vi "CAN_HV_subvi_set.vi"(2 "IP adress HV2":string="1_0_0", 3 "HV Cluster":T1={"HV Power On/Off"=[], "Set Voltage"=[], "HV Tolerance (%)"=1.0}, 4 "IP adress HV1":string="0_0_0") -> (0 "error out":errorcluster, 1 "handle":i32)   [LabVIEW 2012]
uses:
  Program Files/CAEN/HV/CAENHVWrapper/labview/CAENHVWrapper/CAENHVWrapper.lvlib
panel:
  out "Channel On/Off":bool[](array[boolean])
  out "Voltage":string[](array[string])
  out "IP adress used":string
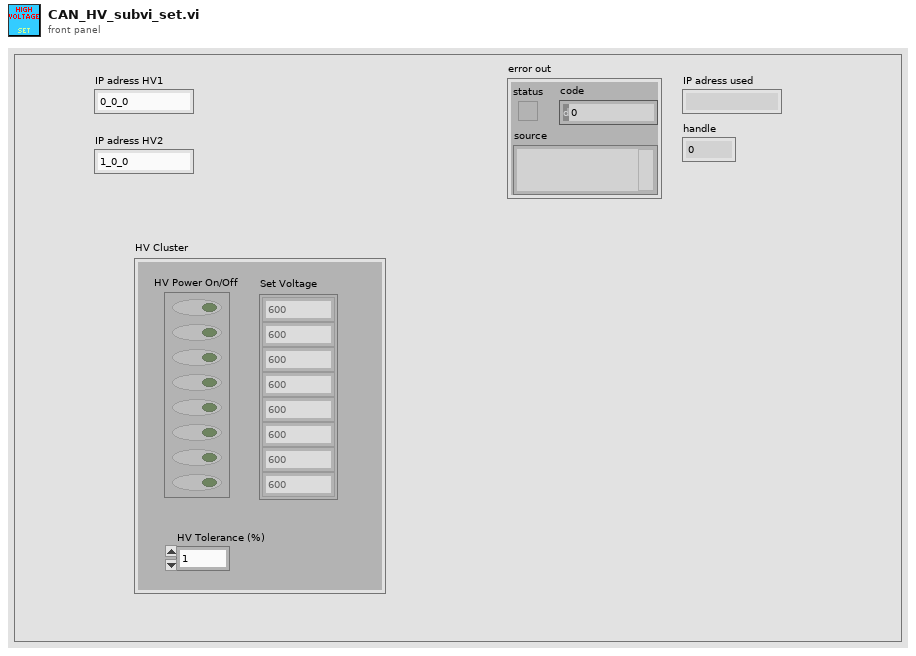
[diagram p1: front panel]
types:
  T1 = cluster{"HV Power On/Off":bool[], "Set Voltage":string[], "HV Tolerance (%)":dbl}
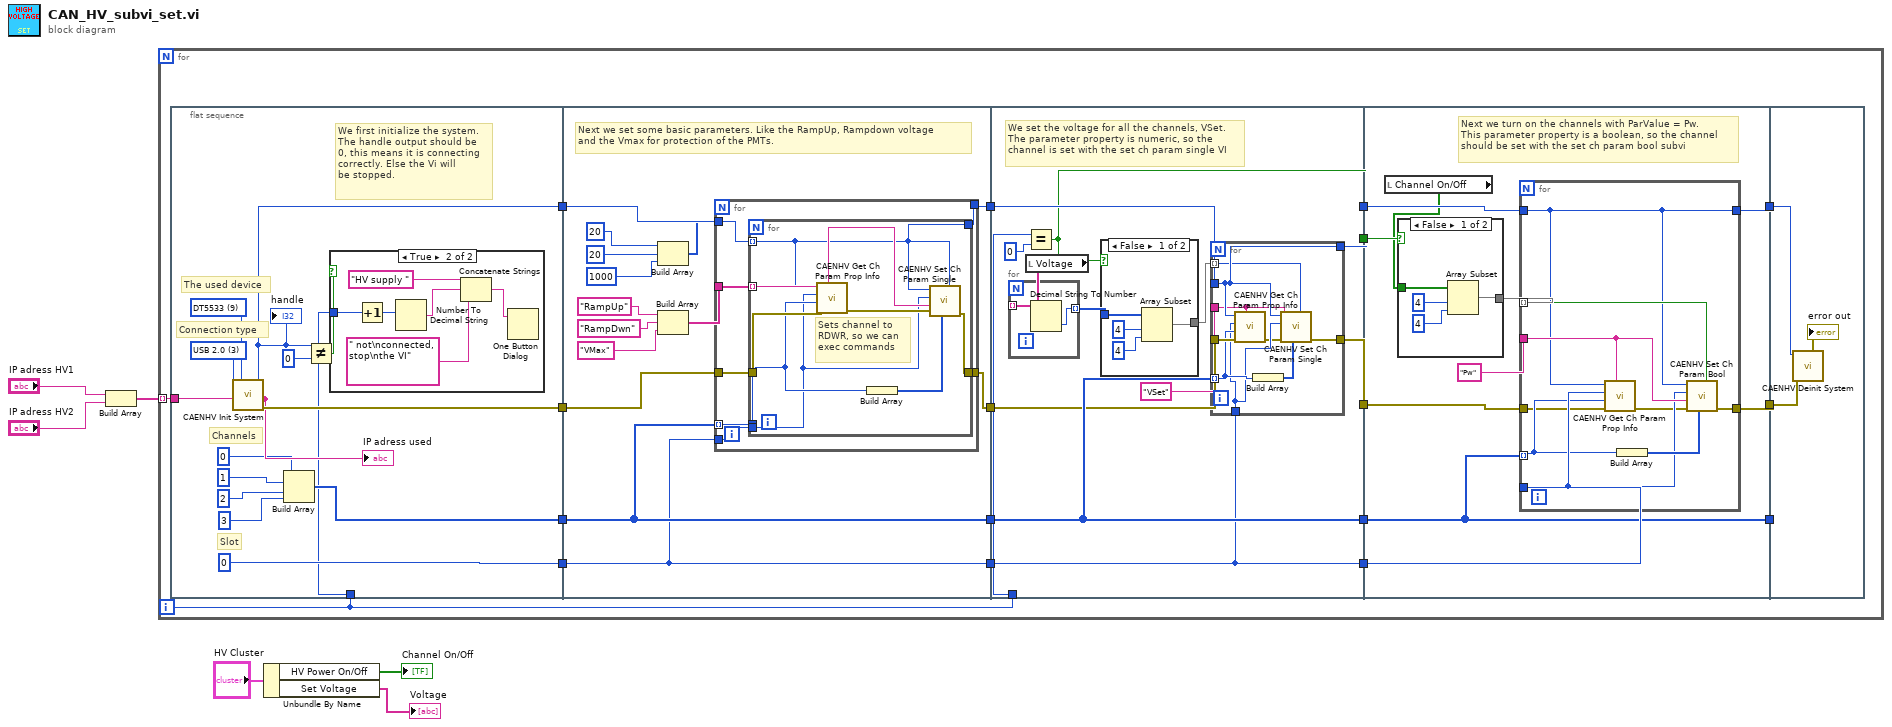
[diagram p0: block diagram]
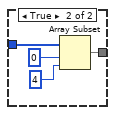
[diagram p3: hidden frame]
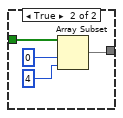
[diagram p4: hidden frame]
diagram:
  n1 = Build Array("IP adress HV1", "IP adress HV2") -> (w4:string[])
  n2 = for {
    tunnel: w4 -> [w12] mode=indexing
    i -> [w7]
    n3 = flat-sequence {
      tunnel: [w36] -> w24
      tunnel: [w32] -> w23
      tunnel: [w33] -> w22
      tunnel: [0] -> w21
      tunnel: w12 -> [w31]
      tunnel: w7 -> [w25]
      tunnel: w24 -> [w56]
      tunnel: w23 -> [w58]
      tunnel: [w57] -> w20
      tunnel: w22 -> [w50]
      tunnel: w21 -> [w49]
      tunnel: [w50] -> w19
      tunnel: [w49] -> w18
      tunnel: [w55] -> w17
      tunnel: w20 -> [w88]
      tunnel: [w87] -> w16
      tunnel: [w84] -> w15
      tunnel: [w86] -> w14
      tunnel: [w85] -> w13
      tunnel: w19 -> [w85]
      tunnel: w18 -> [w84]
      tunnel: w17 -> [w83]
      tunnel: [w79] -> w11
      tunnel: w7 -> [w78]
      tunnel: w16 -> [w116]
      tunnel: w15 -> [w111]
      tunnel: w14 -> [w115]
      tunnel: w13 -> [w110]
      tunnel: w11 -> [w114]
      tunnel: [w113] -> w10
      tunnel: [w112] -> w9
      tunnel: [w110] -> w8
      tunnel: w10 -> [w136]
      tunnel: w9 -> [w135]
      tunnel: w8 -> [_]
      frame #0 {
        w38 = 3 items=["TCP/IP"=0, "HS CAENET"=2, "USB 2.0"=3, "CONET Optical Link"=4, "USB VCP"=5] ("LinkType")
        w37 = u32 9 items=["SY1527", "SY2527", "SY4527", "SY5527", "N568", "V65XX", "N1470", "V8100", "N568E", "DT5533"] ("system")
        # "Connection type"
        # "The used device"
        # "Slot"
        # "Channels"
        # "We first initialize the system.\nThe handle output should be\n0, this means it is connecting\ncorrectly. Else the Vi will\nbe stopped."
        n4 = call "CAENHV Init System.vi"("Arg"=w31, "LinkType"=w38, "system"=w37) -> ("error out"=w36:errorcluster, "handle"=w32:i32)  [unwired: 7 in]
        "handle" <- w32
        n5 = Build Array(0, 1, 2, 3) -> (w33:i32[])
        n6 = Not Equal?(x=w32, y=0) -> (x != y?=w34:bool)
        n7 = case shown="True" w34 {
          tunnel: w25 -> [_ w44]
          frame False {
          }
          frame True {
            n8 = Increment(x=w44) -> (x+1=w43:i32)
            n9 = Number To Decimal String(number=w43) -> (decimal integer string=w41:string)  [unwired: 1 in]
            n10 = Concatenate Strings("HV supply ", w41, " not\nconnected, stop\nthe VI" ("message")) -> (w39:string)
            n11 = One Button Dialog(message=w39) -> ()  [unwired: 1 in, 1 out]
          }
        }
        "IP adress used" <- w31
      }
      frame #1 {
        # "Next we set some basic parameters. Like the RampUp, Rampdown voltage \nand the Vmax for protection of the PMTs."
        n12 = Build Array(20, 20, 1000) -> (w45:i32[])
        n13 = Build Array("RampUp", "RampDwn", "VMax") -> (w51:string[])
        n14 = for {
          tunnel: w58 -> [w61]
          tunnel: [w59] -> w57
          tunnel: w56 -> [w66]
          tunnel: [w65] -> w55
          tunnel: w51 -> [w64]
          tunnel: w50 -> [w63] mode=indexing
          tunnel: w49 -> [w62]
          tunnel: w45 -> [w60]
          n15 = for {
            tunnel: w66 -> [w75]
            tunnel: [w73] -> w65
            tunnel: w64 -> [w71] mode=indexing
            tunnel: w63 -> [w70]
            tunnel: w62 -> [w69]
            tunnel: w61 -> [w67]
            tunnel: w60 -> [w68] mode=indexing
            tunnel: [w67] -> w59
            # "Sets channel to RDWR, so we can exec commands"
            n16 = call "CAENHV Get Ch Param Prop Info.vi"("ParName"=w71, "error in (no error)"=w75, "Ch"=w70, "slot"=w69, "handle"=w67) -> ("error out"=w74:errorcluster)  [unwired: 4 in, 2 out]
            n17 = Build Array(w70) -> (w72:i32[])
            n18 = call "CAENHV Set Ch Param Single.vi"("ParValue"=w68, "ChList"=w72, "error in (no error)"=w74, "ParName"=w71, "slot"=w69, "handle"=w67) -> ("error out"=w73:errorcluster)  [unwired: 5 in]
          }
        }
      }
      frame #2 {
        # "We set the voltage for all the channels, VSet.\nThe parameter property is numeric, so the\nchannel is set with the set ch param single VI"
        n19 = Equal?(x=w78, y=0) -> (x = y?=w79:bool)
        n20 = local read "Voltage"() -> (w77:string[])
        n21 = for {
          tunnel: w77 -> [w90] mode=indexing
          tunnel: [w89] -> w76 mode=indexing
          n22 = Decimal String To Number(string=w90) -> (number=w89:i32)  [unwired: 2 in, 1 out]
        }
        n23 = case shown="False" w79 {
          tunnel: [w91 w96] -> w81
          tunnel: w76 -> [w92 w95]
          frame False {
            n24 = Array Subset(array=w92, index=4, length=4) -> (w91:i32[])
          }
          frame True {
            n25 = Array Subset(array=w95, index=0, length=4) -> (w96:i32[])
          }
        }
        n26 = for {
          tunnel: "VSet" ("Setvoltage") -> [w103]
          tunnel: w83 -> [w107]
          tunnel: w85 -> [w106] mode=indexing
          tunnel: w84 -> [w104]
          tunnel: w88 -> [w105]
          tunnel: [w105] -> w87
          tunnel: [w102] -> w86
          tunnel: w81 -> [w101] mode=indexing
          n27 = call "CAENHV Get Ch Param Prop Info.vi"("ParName"=w103, "error in (no error)"=w107, "Ch"=w106, "slot"=w104, "handle"=w105) -> ("error out"=w99:errorcluster)  [unwired: 4 in, 2 out]
          n28 = Build Array(w106) -> (w100:i32[])
          n29 = call "CAENHV Set Ch Param Single.vi"("ParValue"=w101, "ChList"=w100, "error in (no error)"=w99, "ParName"=w103, "slot"=w104, "handle"=w105) -> ("error out"=w102:errorcluster)  [unwired: 5 in]
        }
      }
      frame #3 {
        # "Next we turn on the channels with ParValue = Pw. \nThis parameter property is a boolean, so the channel\nshould be set with the set ch param bool subvi"
        n30 = local read "Channel On/Off"() -> (w108:bool[])
        n31 = case shown="False" w114 {
          tunnel: [w118 w123] -> w109
          tunnel: w108 -> [w119 w122]
          frame False {
            n32 = Array Subset(array=w119, index=4, length=4) -> (w118:bool[])
          }
          frame True {
            n33 = Array Subset(array=w122, index=0, length=4) -> (w123:bool[])
          }
        }
        n34 = for {
          tunnel: w109 -> [w134] mode=indexing
          tunnel: [w133] -> w112
          tunnel: "Pw" ("ParName") -> [w132]
          tunnel: w116 -> [w130]
          tunnel: [w130] -> w113
          tunnel: w111 -> [w129]
          tunnel: w110 -> [w128] mode=indexing
          tunnel: w115 -> [w127]
          n35 = call "CAENHV Get Ch Param Prop Info.vi"("ParName"=w132, "error in (no error)"=w127, "Ch"=w128, "slot"=w129, "handle"=w130) -> ("error out"=w126:errorcluster)  [unwired: 4 in, 2 out]
          n36 = Build Array(w128) -> (w131:i32[])
          n37 = call "CAENHV Set Ch Param Bool.vi"("ParValue"=w134, "ChList"=w131, "error in (no error)"=w126, "ParName"=w132, "slot"=w129, "handle"=w130) -> ("error out"=w133:errorcluster)  [unwired: 5 in]
        }
      }
      frame #4 {
        n38 = call "CAENHV Deinit System.vi"("error in (no error)"=w135, "handle"=w136) -> ("error out"=→"error out":errorcluster)  [unwired: 9 in]
      }
    }
  }
  n39 = Unbundle By Name("HV Cluster") -> ("HV Power On/Off"=→"Channel On/Off":bool[], "Set Voltage"=→"Voltage":string[])
